vi "magnets-archive.vi"(0 "archive in":T5={"sync"={"elyse/sync/NI6071E/delay"=1.5500000000000005, "elyse/sync/NI6071E/width"=1.0, "elyse/sync/frequency/delay"=10.0, "elyse/sync/frequency/width"=181000.0, "elyse/sync/WCM/delay"=2177.9, "elyse/sync/WCM/width"=10.0, "elyse/sync/modulator/delay"=2182.400000000002, "elyse/sync/modulator/width"=3.0, "elyse/sync/HF/delay"=2175.0, "elyse/sync/HF/width"=3.0, "elyse/sync/Faraday/delay"=5080.0, "elyse/sync/Faraday/width"=100.0, "elyse/sync/Oscilloscope/delay"=2175.0, "elyse/sync/Oscilloscope/width"=2.8, "elyse/sync/50Hz_20MHz/delay"=1.0, "elyse/sync/50Hz_20MHz/width"=5000.0, "elyse/sync/laser_HF/delay"=0.35, "elyse/sync/laser_HF/width"=0.35, "elyse/sync/IMAC/delay"=2176.0, "elyse/sync/IMAC/width"=100.0, "elyse/sync/laser/delay"=2008.3, "elyse/sync/laser/width"=10.0, "elyse/sync/oscilloscope1/delay"=2175.0, "elyse/sync/oscilloscope1/width"=10.0, "elyse/sync/oscilloscope2/delay"=2175.0, "elyse/sync/oscilloscope2/width"=100.0, "elyse/sync/detection1/delay"=500.0, "elyse/sync/detection1/width"=500.0, "elyse/sync/detection1/delay"=0.3, "elyse/sync/detection2/width"=10.0, "elyse/sync/machine/delay"=2175.0, "elyse/sync/machine/width"=100.0, "elyse/sync/n_selection"=4.0}, "HT"={"elyse/HT/voltage/set_value"=6.5, "elyse/HT/voltage/value"=1.5625e-08, "elyse/HT/current/value"=0.0, "elyse/preamplifier/set_value"=1.5625e-08, "elyse/preamplifier/value"=0.0}, "HF"={"elyse/HF/attenuator/value"=-0.01903046052094623, "elyse/HF/dephaser/value"=-18.585806237727724, "elyse/HF/dephaser/value_manuel"=-78.82860725035081, "elyse/HF/canon/value"=0.0, "elyse/HF/section/value"=-18.585806237727724}, "vacuum"={"elyse/vacuum/preparation_chamber/state"=TRUE, "elyse/vacuum/preparation_chamber/measurement"=0.0, "elyse/vacuum/HF/state"=TRUE, "elyse/vacuum/HF/measurement"=0.0, "elyse/vacuum/canon/state"=TRUE, "elyse/vacuum/canon/measurement"=0.0, "elyse/vacuum/section/state"=TRUE, "elyse/vacuum/section/measurement"=0.0, "elyse/vacuum/dipole1/state"=TRUE, "elyse/vacuum/dipole1/measurement"=0.0, "elyse/vacuum/screen1/state"=TRUE, "elyse/vacuum/screen1/measurement"=0.0, "elyse/vacuum/mirror/state"=TRUE, "elyse/vacuum/mirror/measurement"=0.0, "elyse/vacuum/tpg300_section/state"=TRUE, "elyse/vacuum/tpg300_section/measurement"=0.0, "elyse/vacuum/valves/cathode/state"=FALSE, "elyse/vacuum/valves/injection/state"=FALSE}, "modulator"={"elyse/modulator/focale1/current/value"=0.0, "elyse/modulator/focale2/current/value"=0.0, "elyse/modulator/focale3/current/value"=0.0, "elyse/modulator/LAR/voltage/value"=0.0, "elyse/modulator/line_end/current/value"=0.0, "elyse/modulator/thyratron/currents/power/value"=0.0, "elyse/modulator/thyratron_reservoir/current/value"=0.0, "elyse/modulator/paramagnetization/current/value"=0.0, "elyse/modulator/thyratron/voltages/heating/value"=0.0, "elyse/modulator/thyratron/currents/heating/value"=0.0, "elyse/modulator/klystron/currents/power/value"=0.0, "elyse/modulator/klystron/voltages/power/value"=0.0, "elyse/modulator/klystron/currents/heating/value"=0.0, "elyse/modulator/klystron/voltages/heating/value"=0.0}, "cooling"={"elyse/cooling/section/temperature/set_value"=28.0, "elyse/cooling/section/temperature/measurement"=27.96142578125, "elyse/cooling/canon/temperature/set_value"=20.2, "elyse/cooling/canon/temperature/measurement"=26.69921875}, "magnets"={"elyse/magnets/focale/set_value"=0.0, "elyse/magnets/focale/value"=0.0, "elyse/magnets/phase_HF_laser/set_value"=0.0, "elyse/magnets/phase_HF_laser/value"=0.0, "elyse/magnets/dipole1/set_value"=0.0, "elyse/magnets/dipole1/value"=0.0, "elyse/magnets/dipole2/set_value"=0.0, "elyse/magnets/dipole2/value"=0.0, "elyse/magnets/Cor_H1/set_value"=0.0, "elyse/magnets/Cor_H1/value"=0.0, "elyse/magnets/Cor_V1/set_value"=0.0, "elyse/magnets/Cor_V1/value"=0.0, "elyse/magnets/Cor_H2/set_value"=0.0, "elyse/magnets/Cor_H2/value"=0.0, "elyse/magnets/Cor_V2/set_value"=0.0, "elyse/magnets/Cor_V2/value"=0.0, "elyse/magnets/Cor_H3/set_value"=0.0, "elyse/magnets/Cor_H3/value"=0.0, "elyse/magnets/Cor_V3/set_value"=-5.0, "elyse/magnets/Cor_V3/value"=0.0, "elyse/magnets/Cor_H4/set_value"=0.0, "elyse/magnets/Cor_H4/value"=0.0, "elyse/magnets/Cor_V4/set_value"=0.0, "elyse/magnets/Cor_V4/value"=0.0, "elyse/magnets/Cor_H5/set_value"=0.0, "elyse/magnets/Cor_H5/value"=0.0, "elyse/magnets/Cor_V5/set_value"=0.0, "elyse/magnets/Cor_V5/value"=0.0, "elyse/magnets/triplet1-1/set_value"=0.0, "elyse/magnets/triplet1-1/value"=0.0, "elyse/magnets/triplet1-2/set_value"=0.0, "elyse/magnets/triplet1-2/value"=0.0, "elyse/magnets/triplet2-1/set_value"=0.0, "elyse/magnets/triplet2-1/value"=0.0, "elyse/magnets/triplet2-2/set_value"=0.0, "elyse/magnets/triplet2-2/value"=0.0, "elyse/magnets/qudrupole1/set_value"=0.0, "elyse/magnets/qudrupole1/value"=0.0, "elyse/magnets/qudrupole2/set_value"=0.0, "elyse/magnets/qudrupole2/value"=0.0}, "time"={"elyse/timestamp"=0.0}}, 1 "C6NI6703":T3 {"09 OUT09 b37 Cmd Guidage V5" format="%.3f"; "08 OUT08 b33 Réserve" format="%.3f"; "07 OUT07 b29 Cmd Guidage V4" format="%.3f"; "06 OUT06 b25 Cmd Guidage H4" format="%.3f"; "05 OUT05 b21 Cmd Guidage V3" format="%.3f"; "04 OUT04 b17 Cmd Guidage H3" format="%.3f"; "03 OUT03 b13 Cmd Guidage V2" format="%.3f"; "02 OUT02 b09 Cmd Guidage H2" format="%.3f"; "01 OUT01 b05 Cmd Guidage V1" format="%.3f"; "00 OUT00 b01 Cmd Guidage H1" format="%.3f"}, 2 "C7NI6703":T2 {"09 OUT09 b37 Cmd I Dipôle 2" format="%.3f"; "08 OUT08 b33 Cmd I Dipôle 1" format="%.3f"; "07 OUT07 b29 Cmd I Quad 2" format="%.3f"; "06 OUT06 b25 Cmd I Quad 1" format="%.3f"; "05 OUT05 b21 Cmd I Solénoïde" format="%.3f"; "04 OUT04 b17 Cmd I Triplet 2-2" format="%.3f"; "03 OUT03 b13 Cmd I Triplet 2-1" format="%.3f"; "02 OUT02 b09 Réserve" format="%.3f"; "01 OUT01 b05 Cmd I Triplet 1-2" format="%.3f"; "00 OUT00 b01 Cmd I Triplet 1-1" format="%.3f"}, 3 "C8NI6703":T4 {"09 OUT09 b37 Cmd position Miroir Y" format="%.3f"; "08 OUT08 b33 Cmd position Miroir X" format="%.3f"; "07 OUT07 b29 Réserve" format="%.3f"; "06 OUT06 b25 Cmd amplitude HF préampli" format="%.3f"; "05 OUT05 b21 Cmd déphasage HF/LASER" format="%.3f"; "04 OUT04 b17 Cmd Pos. Atténuateur" format="%.3f"; "03 OUT03 b13 Cmd Pos. Déphaseur" format="%.3f"; "02 OUT02 b09 Cmd Temp. Section" format="%.3f"; "01 OUT01 b05 Cmd Temp. Canon" format="%.3f"; "00 OUT00 b01 Réserve" format="%.3f"}, 4 "C1NI6071E":T1 {"63 ACH63 b100 Libre ?" format="%.3f"; "62 ACH62 b98 Libre ?" format="%.3f"; "61 ACH61 b96 Libre ?" format="%.3f"; "60 ACH60 b94 Libre ?" format="%.3f"; "59 ACH59 b92 Libre ?" format="%.3f"; "58 ACH58 b90 Libre ?" format="%.3f"; "57 ACH57 b88 Libre ?" format="%.3f"; "56 ACH56 b86 Libre ?" format="%.3f"; "55 ACH55 b99 Libre ?" format="%.3f"; "54 ACH54 b97 Libre ?" format="%.3f"; "53 ACH53 b95 Libre ?" format="%.3f"; "52 ACH52 b93 Libre ?" format="%.3f"; "51 ACH51 b91 Libre ?" format="%.3f"; "50 ACH50 b89 Libre ?" format="%.3f"; "49 ACH49 b87 Libre ?" format="%.3f"; "48 ACH48 b85 Réservé" format="%.3f"; "47 ACH47 b84 Réservé" format="%.3f"; "46 ACH46 b82 Réservé" format="%.3f"; "45 ACH45 b80 Mesure phase HF1" format="%.3f"; "44 ACH44 b78 Mesure Atténuateur" format="%.3f"; "43 ACH43 b74 Réservé" format="%.3f"; "42 ACH42 b72 Mes champ Dipôle 2" format="%.3f"; "41 ACH41 b70 Mes H5" format="%.3f"; "40 ACH40 b68 Mes I correcte Dipôle 21 (H4)" format="%.3f"; "39 ACH39 b83 Réservé" format="%.3f"; "38 ACH38 b81 Mesure phase HF2" format="%.3f"; "37 ACH37 b79 Mes position Déphaseur ajust" format="%.3f"; "36 ACH36 b77 Mes position Déphaseur" format="%.3f"; "35 ACH35 b73 Mes champ Dipôle 2" format="%.3f"; "34 ACH34 b71 Mes I Guidage V5" format="%.3f"; "33 ACH33 b69 Mes I Guidage V4" format="%.3f"; "32 ACH32 b67 Mes I Guidage V3" format="%.3f"; "31 ACH31 b66 Mes I correcte Dipôle 1 (H3)" format="%.3f"; "30 ACH30 b64 Mes I Guidage H2" format="%.3f"; "29 ACH29 b62 Mes I Guidage H1" format="%.3f"; "28 ACH28 b60 Mes I Dipôle 1" format="%.3f"; "27 ACH27 b58 Mes I Quadripôle 2" format="%.3f"; "26 ACH26 b56 Réservé" format="%.3f"; "25 ACH25 b54 Mes I Triplet 2-1" format="%.3f"; "24 ACH24 b52 Mes I Triplet 1-2" format="%.3f"; "23 ACH23 b65 Mes I Guidage V2" format="%.3f"; "22 ACH22 b63 Mes I Guidage V1" format="%.3f"; "21 ACH21 b61 Mes I Dipôle 2" format="%.3f"; "20 ACH20 b59 Mes I Solénoïde" format="%.3f"; "19 ACH19 b57 Mes I Quadripôle 1" format="%.3f"; "18 ACH18 b55 Mes I Triplet 2-2" format="%.3f"; "17 ACH17 b53 Réservé" format="%.3f"; "16 ACH16 b51 Mes I Triplet 1-1" format="%.3f"; "15 ACH15 b18 Libre ?" format="%.3f"; "14 ACH14 b16 Libre ?" format="%.3f"; "13 ACH13 b14 Libre ?" format="%.3f"; "12 ACH12 b12 Mes Vide jauge canon" format="%.3f"; "11 ACH11 b10 Mes Vide DIP 1 (PIQ27 + 33)" format="%.3f"; "10 ACH10 b08 Mes Vide Section (PIQ 16)" format="%.3f"; "09 ACH09 b06 Mes Vide SAS guide HF" format="%.3f"; "08 ACH08 b04 Mes température Section" format="%.3f"; "07 ACH07 b17 Libre ?" format="%.3f"; "06 ACH06 b15 Libre ?" format="%.3f"; "05 ACH05 b13 Libre ?" format="%.3f"; "04 ACH04 b11 Mes Vide Ecran 1 (PIQ 53-63)" format="%.3f"; "03 ACH03 b09 Mes Vide Miroir (PIQ 21)" format="%.3f"; "02 ACH02 b07 Mes Vide Canon (PIQ 12)" format="%.3f"; "01 ACH01 b05 Mes Vide Chambre de préparation" format="%.3f"; "00 ACH00 b03 Mes température Canon" format="%.3f"}) -> (5 "archive out":T5={"sync"={"elyse/sync/NI6071E/delay"=1.5500000000000005, "elyse/sync/NI6071E/width"=1.0, "elyse/sync/frequency/delay"=10.0, "elyse/sync/frequency/width"=181000.0, "elyse/sync/WCM/delay"=2177.9, "elyse/sync/WCM/width"=10.0, "elyse/sync/modulator/delay"=2182.400000000002, "elyse/sync/modulator/width"=3.0, "elyse/sync/HF/delay"=2175.0, "elyse/sync/HF/width"=3.0, "elyse/sync/Faraday/delay"=5080.0, "elyse/sync/Faraday/width"=100.0, "elyse/sync/Oscilloscope/delay"=2175.0, "elyse/sync/Oscilloscope/width"=2.8, "elyse/sync/50Hz_20MHz/delay"=1.0, "elyse/sync/50Hz_20MHz/width"=5000.0, "elyse/sync/laser_HF/delay"=0.35, "elyse/sync/laser_HF/width"=0.35, "elyse/sync/IMAC/delay"=2176.0, "elyse/sync/IMAC/width"=100.0, "elyse/sync/laser/delay"=2008.3, "elyse/sync/laser/width"=10.0, "elyse/sync/oscilloscope1/delay"=2175.0, "elyse/sync/oscilloscope1/width"=10.0, "elyse/sync/oscilloscope2/delay"=2175.0, "elyse/sync/oscilloscope2/width"=100.0, "elyse/sync/detection1/delay"=500.0, "elyse/sync/detection1/width"=500.0, "elyse/sync/detection1/delay"=0.3, "elyse/sync/detection2/width"=10.0, "elyse/sync/machine/delay"=2175.0, "elyse/sync/machine/width"=100.0, "elyse/sync/n_selection"=4.0}, "HT"={"elyse/HT/voltage/set_value"=6.5, "elyse/HT/voltage/value"=1.5625e-08, "elyse/HT/current/value"=0.0, "elyse/preamplifier/set_value"=1.5625e-08, "elyse/preamplifier/value"=0.0}, "HF"={"elyse/HF/attenuator/value"=-0.01903046052094623, "elyse/HF/dephaser/value"=-18.585806237727724, "elyse/HF/dephaser/value_manuel"=-78.82860725035081, "elyse/HF/canon/value"=0.0, "elyse/HF/section/value"=-18.585806237727724}, "vacuum"={"elyse/vacuum/preparation_chamber/state"=TRUE, "elyse/vacuum/preparation_chamber/measurement"=0.0, "elyse/vacuum/HF/state"=TRUE, "elyse/vacuum/HF/measurement"=0.0, "elyse/vacuum/canon/state"=TRUE, "elyse/vacuum/canon/measurement"=0.0, "elyse/vacuum/section/state"=TRUE, "elyse/vacuum/section/measurement"=0.0, "elyse/vacuum/dipole1/state"=TRUE, "elyse/vacuum/dipole1/measurement"=0.0, "elyse/vacuum/screen1/state"=TRUE, "elyse/vacuum/screen1/measurement"=0.0, "elyse/vacuum/mirror/state"=TRUE, "elyse/vacuum/mirror/measurement"=0.0, "elyse/vacuum/tpg300_section/state"=TRUE, "elyse/vacuum/tpg300_section/measurement"=0.0, "elyse/vacuum/valves/cathode/state"=FALSE, "elyse/vacuum/valves/injection/state"=FALSE}, "modulator"={"elyse/modulator/focale1/current/value"=0.0, "elyse/modulator/focale2/current/value"=0.0, "elyse/modulator/focale3/current/value"=0.0, "elyse/modulator/LAR/voltage/value"=0.0, "elyse/modulator/line_end/current/value"=0.0, "elyse/modulator/thyratron/currents/power/value"=0.0, "elyse/modulator/thyratron_reservoir/current/value"=0.0, "elyse/modulator/paramagnetization/current/value"=0.0, "elyse/modulator/thyratron/voltages/heating/value"=0.0, "elyse/modulator/thyratron/currents/heating/value"=0.0, "elyse/modulator/klystron/currents/power/value"=0.0, "elyse/modulator/klystron/voltages/power/value"=0.0, "elyse/modulator/klystron/currents/heating/value"=0.0, "elyse/modulator/klystron/voltages/heating/value"=0.0}, "cooling"={"elyse/cooling/section/temperature/set_value"=28.0, "elyse/cooling/section/temperature/measurement"=27.96142578125, "elyse/cooling/canon/temperature/set_value"=20.2, "elyse/cooling/canon/temperature/measurement"=26.69921875}, "magnets"={"elyse/magnets/focale/set_value"=0.0, "elyse/magnets/focale/value"=0.0, "elyse/magnets/phase_HF_laser/set_value"=0.0, "elyse/magnets/phase_HF_laser/value"=0.0, "elyse/magnets/dipole1/set_value"=0.0, "elyse/magnets/dipole1/value"=0.0, "elyse/magnets/dipole2/set_value"=0.0, "elyse/magnets/dipole2/value"=0.0, "elyse/magnets/Cor_H1/set_value"=0.0, "elyse/magnets/Cor_H1/value"=0.0, "elyse/magnets/Cor_V1/set_value"=0.0, "elyse/magnets/Cor_V1/value"=0.0, "elyse/magnets/Cor_H2/set_value"=0.0, "elyse/magnets/Cor_H2/value"=0.0, "elyse/magnets/Cor_V2/set_value"=0.0, "elyse/magnets/Cor_V2/value"=0.0, "elyse/magnets/Cor_H3/set_value"=0.0, "elyse/magnets/Cor_H3/value"=0.0, "elyse/magnets/Cor_V3/set_value"=-5.0, "elyse/magnets/Cor_V3/value"=0.0, "elyse/magnets/Cor_H4/set_value"=0.0, "elyse/magnets/Cor_H4/value"=0.0, "elyse/magnets/Cor_V4/set_value"=0.0, "elyse/magnets/Cor_V4/value"=0.0, "elyse/magnets/Cor_H5/set_value"=0.0, "elyse/magnets/Cor_H5/value"=0.0, "elyse/magnets/Cor_V5/set_value"=0.0, "elyse/magnets/Cor_V5/value"=0.0, "elyse/magnets/triplet1-1/set_value"=0.0, "elyse/magnets/triplet1-1/value"=0.0, "elyse/magnets/triplet1-2/set_value"=0.0, "elyse/magnets/triplet1-2/value"=0.0, "elyse/magnets/triplet2-1/set_value"=0.0, "elyse/magnets/triplet2-1/value"=0.0, "elyse/magnets/triplet2-2/set_value"=0.0, "elyse/magnets/triplet2-2/value"=0.0, "elyse/magnets/qudrupole1/set_value"=0.0, "elyse/magnets/qudrupole1/value"=0.0, "elyse/magnets/qudrupole2/set_value"=0.0, "elyse/magnets/qudrupole2/value"=0.0}, "time"={"elyse/timestamp"=0.0}})   [LabVIEW 2020]
uses:
  archive.ctl
  sync_type_def.ctl
  HT_type-def.ctl
  HF_type_def.ctl
  vacuum_type_def.ctl
  modulator_type_def.ctl
  water_cooling_type_def.ctl
  all_magnets_type_def.ctl
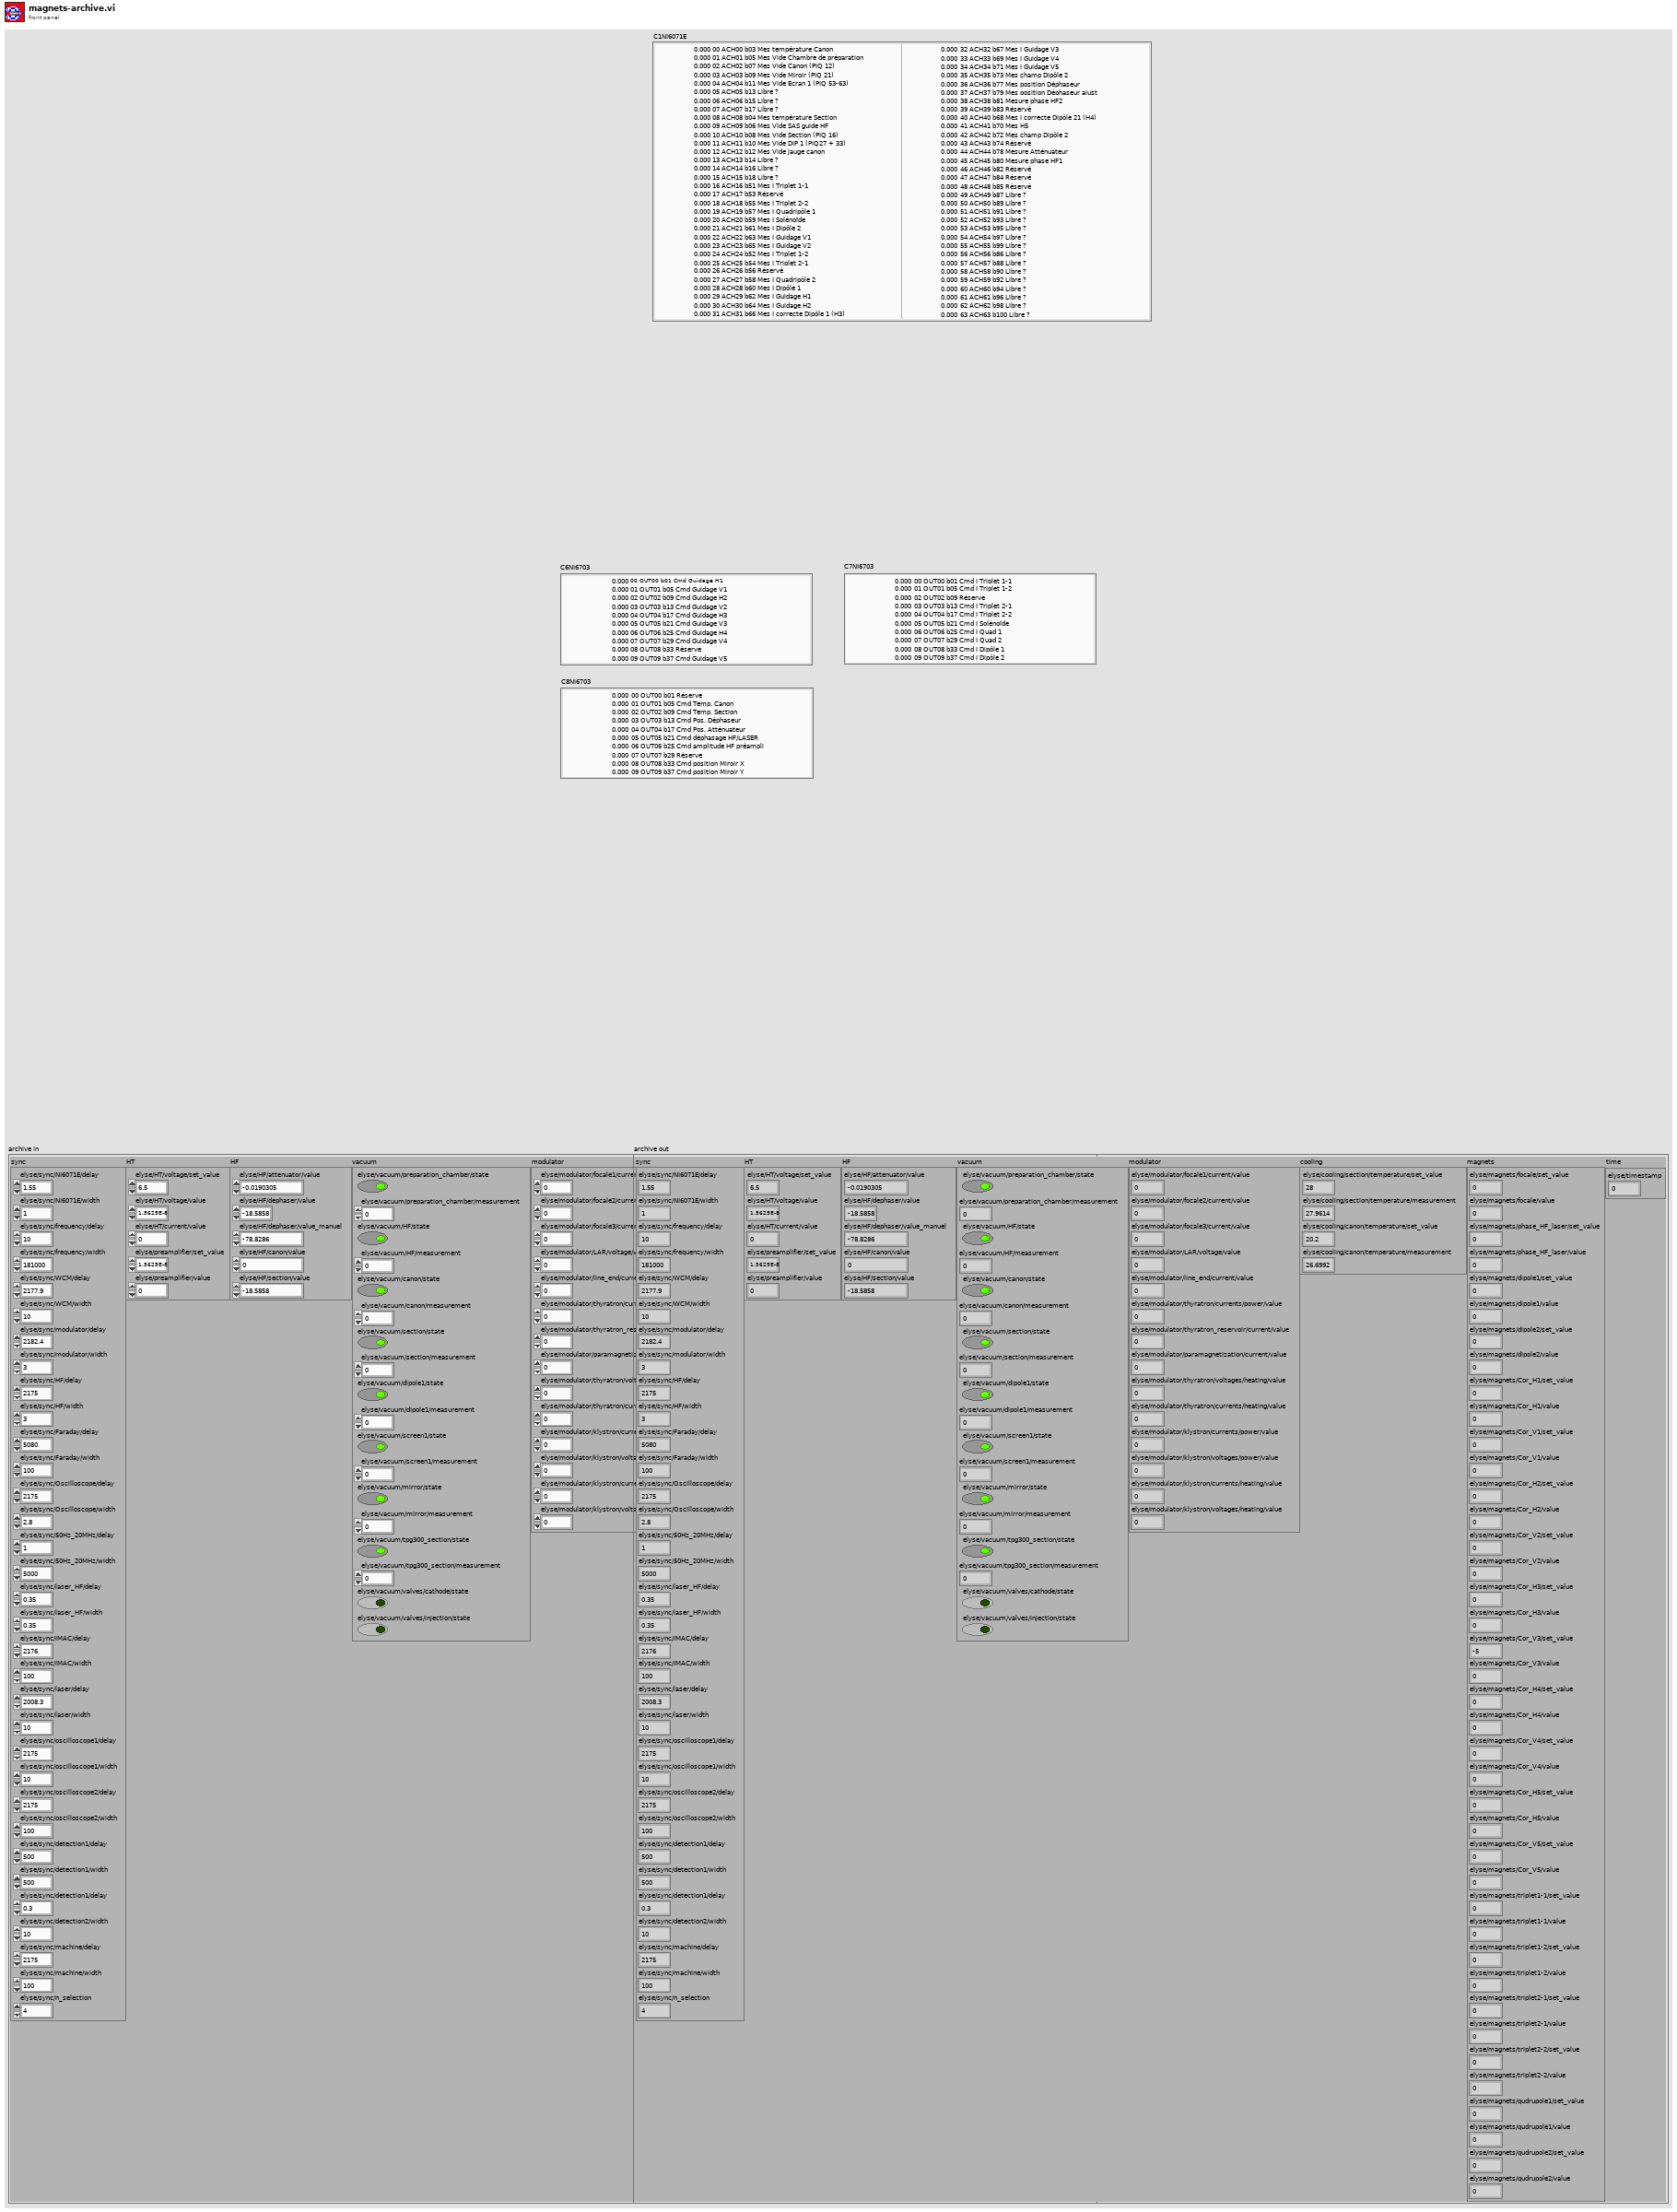
[diagram p1: front panel]
types:
  T1 = cluster{"00 ACH00 b03 Mes température Canon":dbl, "01 ACH01 b05 Mes Vide Chambre de préparation":dbl, "02 ACH02 b07 Mes Vide Canon (PIQ 12)":dbl, "03 ACH03 b09 Mes Vide Miroir (PIQ 21)":dbl, "04 ACH04 b11 Mes Vide Ecran 1 (PIQ 53-63)":dbl, "05 ACH05 b13 Libre ?":dbl, "06 ACH06 b15 Libre ?":dbl, "07 ACH07 b17 Libre ?":dbl, "08 ACH08 b04 Mes température Section":dbl, "09 ACH09 b06 Mes Vide SAS guide HF":dbl, "10 ACH10 b08 Mes Vide Section (PIQ 16)":dbl, "11 ACH11 b10 Mes Vide DIP 1 (PIQ27 + 33)":dbl, "12 ACH12 b12 Mes Vide jauge canon":dbl, "13 ACH13 b14 Libre ?":dbl, "14 ACH14 b16 Libre ?":dbl, "15 ACH15 b18 Libre ?":dbl, "16 ACH16 b51 Mes I Triplet 1-1":dbl, "17 ACH17 b53 Réservé":dbl, "18 ACH18 b55 Mes I Triplet 2-2":dbl, "19 ACH19 b57 Mes I Quadripôle 1":dbl, "20 ACH20 b59 Mes I Solénoïde":dbl, "21 ACH21 b61 Mes I Dipôle 2":dbl, "22 ACH22 b63 Mes I Guidage V1":dbl, "23 ACH23 b65 Mes I Guidage V2":dbl, "24 ACH24 b52 Mes I Triplet 1-2":dbl, "25 ACH25 b54 Mes I Triplet 2-1":dbl, "26 ACH26 b56 Réservé":dbl, "27 ACH27 b58 Mes I Quadripôle 2":dbl, "28 ACH28 b60 Mes I Dipôle 1":dbl, "29 ACH29 b62 Mes I Guidage H1":dbl, "30 ACH30 b64 Mes I Guidage H2":dbl, "31 ACH31 b66 Mes I correcte Dipôle 1 (H3)":dbl, "32 ACH32 b67 Mes I Guidage V3":dbl, "33 ACH33 b69 Mes I Guidage V4":dbl, "34 ACH34 b71 Mes I Guidage V5":dbl, "35 ACH35 b73 Mes champ Dipôle 2":dbl, "36 ACH36 b77 Mes position Déphaseur":dbl, "37 ACH37 b79 Mes position Déphaseur ajust":dbl, "38 ACH38 b81 Mesure phase HF2":dbl, "39 ACH39 b83 Réservé":dbl, "40 ACH40 b68 Mes I correcte Dipôle 21 (H4)":dbl, "41 ACH41 b70 Mes H5":dbl, "42 ACH42 b72 Mes champ Dipôle 2":dbl, "43 ACH43 b74 Réservé":dbl, "44 ACH44 b78 Mesure Atténuateur":dbl, "45 ACH45 b80 Mesure phase HF1":dbl, "46 ACH46 b82 Réservé":dbl, "47 ACH47 b84 Réservé":dbl, "48 ACH48 b85 Réservé":dbl, "49 ACH49 b87 Libre ?":dbl, "50 ACH50 b89 Libre ?":dbl, "51 ACH51 b91 Libre ?":dbl, "52 ACH52 b93 Libre ?":dbl, "53 ACH53 b95 Libre ?":dbl, "54 ACH54 b97 Libre ?":dbl, "55 ACH55 b99 Libre ?":dbl, "56 ACH56 b86 Libre ?":dbl, "57 ACH57 b88 Libre ?":dbl, "58 ACH58 b90 Libre ?":dbl, "59 ACH59 b92 Libre ?":dbl, "60 ACH60 b94 Libre ?":dbl, "61 ACH61 b96 Libre ?":dbl, "62 ACH62 b98 Libre ?":dbl, "63 ACH63 b100 Libre ?":dbl}
  T2 = cluster{"00 OUT00 b01 Cmd I Triplet 1-1":dbl, "01 OUT01 b05 Cmd I Triplet 1-2":dbl, "02 OUT02 b09 Réserve":dbl, "03 OUT03 b13 Cmd I Triplet 2-1":dbl, "04 OUT04 b17 Cmd I Triplet 2-2":dbl, "05 OUT05 b21 Cmd I Solénoïde":dbl, "06 OUT06 b25 Cmd I Quad 1":dbl, "07 OUT07 b29 Cmd I Quad 2":dbl, "08 OUT08 b33 Cmd I Dipôle 1":dbl, "09 OUT09 b37 Cmd I Dipôle 2":dbl}
  T3 = cluster{"00 OUT00 b01 Cmd Guidage H1":dbl, "01 OUT01 b05 Cmd Guidage V1":dbl, "02 OUT02 b09 Cmd Guidage H2":dbl, "03 OUT03 b13 Cmd Guidage V2":dbl, "04 OUT04 b17 Cmd Guidage H3":dbl, "05 OUT05 b21 Cmd Guidage V3":dbl, "06 OUT06 b25 Cmd Guidage H4":dbl, "07 OUT07 b29 Cmd Guidage V4":dbl, "08 OUT08 b33 Réserve":dbl, "09 OUT09 b37 Cmd Guidage V5":dbl}
  T4 = cluster{"00 OUT00 b01 Réserve":dbl, "01 OUT01 b05 Cmd Temp. Canon":dbl, "02 OUT02 b09 Cmd Temp. Section":dbl, "03 OUT03 b13 Cmd Pos. Déphaseur":dbl, "04 OUT04 b17 Cmd Pos. Atténuateur":dbl, "05 OUT05 b21 Cmd déphasage HF/LASER":dbl, "06 OUT06 b25 Cmd amplitude HF préampli":dbl, "07 OUT07 b29 Réserve":dbl, "08 OUT08 b33 Cmd position Miroir X":dbl, "09 OUT09 b37 Cmd position Miroir Y":dbl}
  T5 = typedef "archive.ctl" = cluster{"sync":T6, "HT":T7, "HF":T8, "vacuum":T9, "modulator":T10, "cooling":T11, "magnets":T12, "time":cluster{"elyse/timestamp":dbl}}
  T6 = typedef "sync_type_def.ctl" = cluster{"elyse/sync/NI6071E/delay":dbl, "elyse/sync/NI6071E/width":dbl, "elyse/sync/frequency/delay":dbl, "elyse/sync/frequency/width":dbl, "elyse/sync/WCM/delay":dbl, "elyse/sync/WCM/width":dbl, "elyse/sync/modulator/delay":dbl, "elyse/sync/modulator/width":dbl, "elyse/sync/HF/delay":dbl, "elyse/sync/HF/width":dbl, "elyse/sync/Faraday/delay":dbl, "elyse/sync/Faraday/width":dbl, "elyse/sync/Oscilloscope/delay":dbl, "elyse/sync/Oscilloscope/width":dbl, "elyse/sync/50Hz_20MHz/delay":dbl, "elyse/sync/50Hz_20MHz/width":dbl, "elyse/sync/laser_HF/delay":dbl, "elyse/sync/laser_HF/width":dbl, "elyse/sync/IMAC/delay":dbl, "elyse/sync/IMAC/width":dbl, "elyse/sync/laser/delay":dbl, "elyse/sync/laser/width":dbl, "elyse/sync/oscilloscope1/delay":dbl, "elyse/sync/oscilloscope1/width":dbl, "elyse/sync/oscilloscope2/delay":dbl, "elyse/sync/oscilloscope2/width":dbl, "elyse/sync/detection1/delay":dbl, "elyse/sync/detection1/width":dbl, "elyse/sync/detection1/delay":dbl, "elyse/sync/detection2/width":dbl, "elyse/sync/machine/delay":dbl, "elyse/sync/machine/width":dbl, "elyse/sync/n_selection":dbl}
  T7 = typedef "HT_type-def.ctl" = cluster{"elyse/HT/voltage/set_value":dbl, "elyse/HT/voltage/value":dbl, "elyse/HT/current/value":dbl, "elyse/preamplifier/set_value":dbl, "elyse/preamplifier/value":dbl}
  T8 = typedef "HF_type_def.ctl" = cluster{"elyse/HF/attenuator/value":dbl, "elyse/HF/dephaser/value":dbl, "elyse/HF/dephaser/value_manuel":dbl, "elyse/HF/canon/value":dbl, "elyse/HF/section/value":dbl}
  T9 = typedef "vacuum_type_def.ctl" = cluster{"elyse/vacuum/preparation_chamber/state":bool, "elyse/vacuum/preparation_chamber/measurement":dbl, "elyse/vacuum/HF/state":bool, "elyse/vacuum/HF/measurement":dbl, "elyse/vacuum/canon/state":bool, "elyse/vacuum/canon/measurement":dbl, "elyse/vacuum/section/state":bool, "elyse/vacuum/section/measurement":dbl, "elyse/vacuum/dipole1/state":bool, "elyse/vacuum/dipole1/measurement":dbl, "elyse/vacuum/screen1/state":bool, "elyse/vacuum/screen1/measurement":dbl, "elyse/vacuum/mirror/state":bool, "elyse/vacuum/mirror/measurement":dbl, "elyse/vacuum/tpg300_section/state":bool, "elyse/vacuum/tpg300_section/measurement":dbl, "elyse/vacuum/valves/cathode/state":bool, "elyse/vacuum/valves/injection/state":bool}
  T10 = typedef "modulator_type_def.ctl" = cluster{"elyse/modulator/focale1/current/value":dbl, "elyse/modulator/focale2/current/value":dbl, "elyse/modulator/focale3/current/value":dbl, "elyse/modulator/LAR/voltage/value":dbl, "elyse/modulator/line_end/current/value":dbl, "elyse/modulator/thyratron/currents/power/value":dbl, "elyse/modulator/thyratron_reservoir/current/value":dbl, "elyse/modulator/paramagnetization/current/value":dbl, "elyse/modulator/thyratron/voltages/heating/value":dbl, "elyse/modulator/thyratron/currents/heating/value":dbl, "elyse/modulator/klystron/currents/power/value":dbl, "elyse/modulator/klystron/voltages/power/value":dbl, "elyse/modulator/klystron/currents/heating/value":dbl, "elyse/modulator/klystron/voltages/heating/value":dbl}
  T11 = typedef "water_cooling_type_def.ctl" = cluster{"elyse/cooling/section/temperature/set_value":dbl, "elyse/cooling/section/temperature/measurement":dbl, "elyse/cooling/canon/temperature/set_value":dbl, "elyse/cooling/canon/temperature/measurement":dbl}
  T12 = typedef "all_magnets_type_def.ctl" = cluster{"elyse/magnets/focale/set_value":dbl, "elyse/magnets/focale/value":dbl, "elyse/magnets/phase_HF_laser/set_value":dbl, "elyse/magnets/phase_HF_laser/value":dbl, "elyse/magnets/dipole1/set_value":dbl, "elyse/magnets/dipole1/value":dbl, "elyse/magnets/dipole2/set_value":dbl, "elyse/magnets/dipole2/value":dbl, "elyse/magnets/Cor_H1/set_value":dbl, "elyse/magnets/Cor_H1/value":dbl, "elyse/magnets/Cor_V1/set_value":dbl, "elyse/magnets/Cor_V1/value":dbl, "elyse/magnets/Cor_H2/set_value":dbl, "elyse/magnets/Cor_H2/value":dbl, "elyse/magnets/Cor_V2/set_value":dbl, "elyse/magnets/Cor_V2/value":dbl, "elyse/magnets/Cor_H3/set_value":dbl, "elyse/magnets/Cor_H3/value":dbl, "elyse/magnets/Cor_V3/set_value":dbl, "elyse/magnets/Cor_V3/value":dbl, "elyse/magnets/Cor_H4/set_value":dbl, "elyse/magnets/Cor_H4/value":dbl, "elyse/magnets/Cor_V4/set_value":dbl, "elyse/magnets/Cor_V4/value":dbl, "elyse/magnets/Cor_H5/set_value":dbl, "elyse/magnets/Cor_H5/value":dbl, "elyse/magnets/Cor_V5/set_value":dbl, "elyse/magnets/Cor_V5/value":dbl, "elyse/magnets/triplet1-1/set_value":dbl, "elyse/magnets/triplet1-1/value":dbl, "elyse/magnets/triplet1-2/set_value":dbl, "elyse/magnets/triplet1-2/value":dbl, "elyse/magnets/triplet2-1/set_value":dbl, "elyse/magnets/triplet2-1/value":dbl, "elyse/magnets/triplet2-2/set_value":dbl, "elyse/magnets/triplet2-2/value":dbl, "elyse/magnets/qudrupole1/set_value":dbl, "elyse/magnets/qudrupole1/value":dbl, "elyse/magnets/qudrupole2/set_value":dbl, "elyse/magnets/qudrupole2/value":dbl}
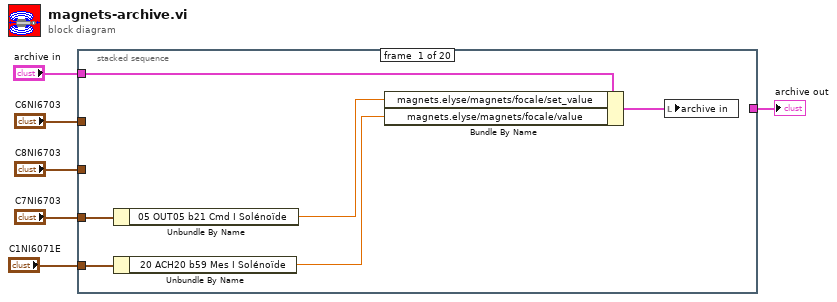
[diagram p0: block diagram]
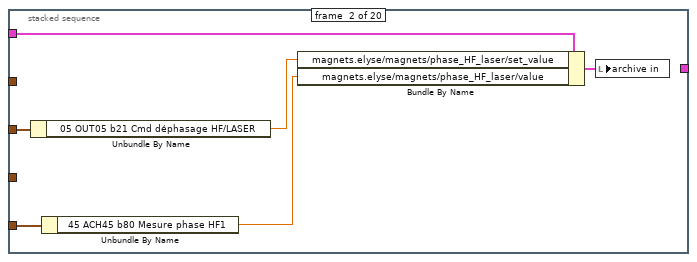
[diagram p2: hidden frame]
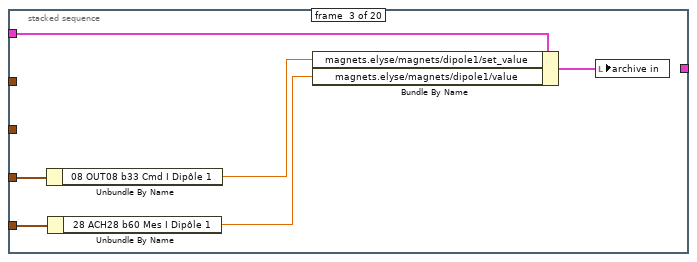
[diagram p3: hidden frame]
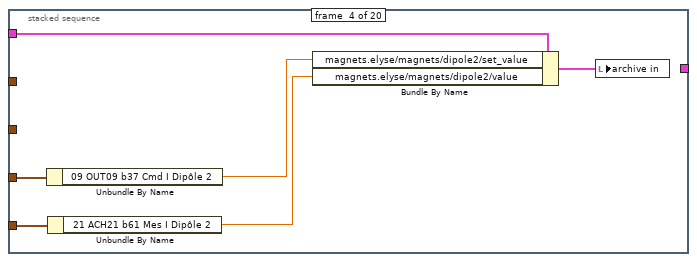
[diagram p4: hidden frame]
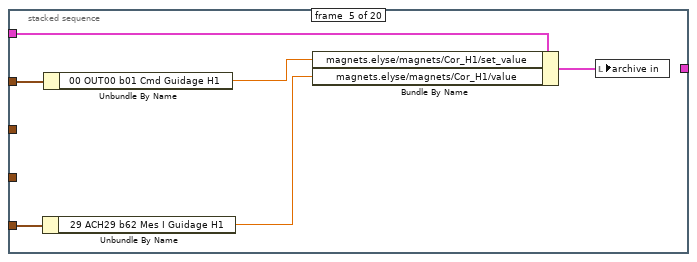
[diagram p5: hidden frame]
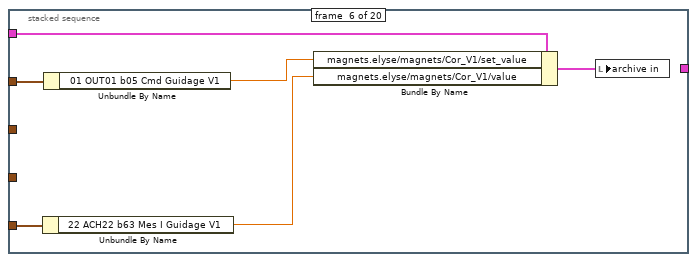
[diagram p6: hidden frame]
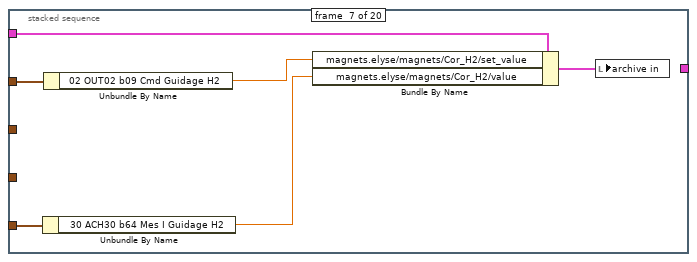
[diagram p7: hidden frame]
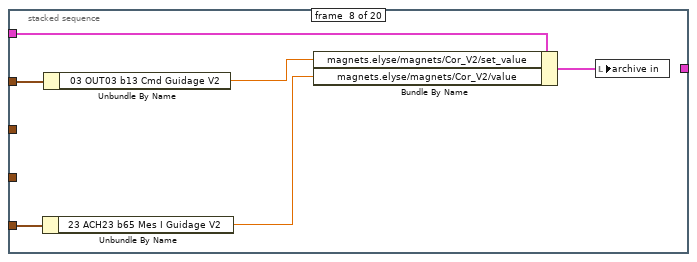
[diagram p8: hidden frame]
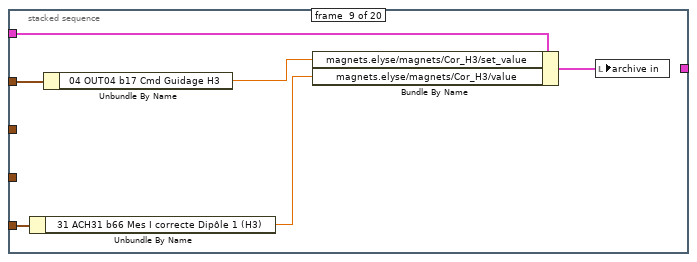
[diagram p9: hidden frame]
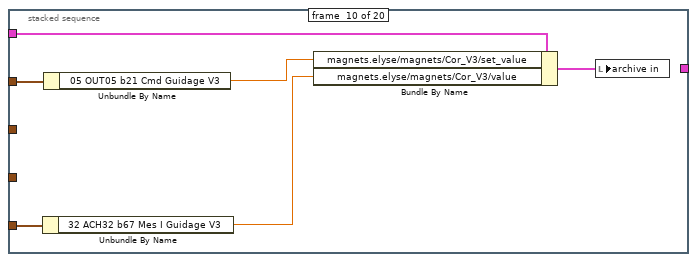
[diagram p10: hidden frame]
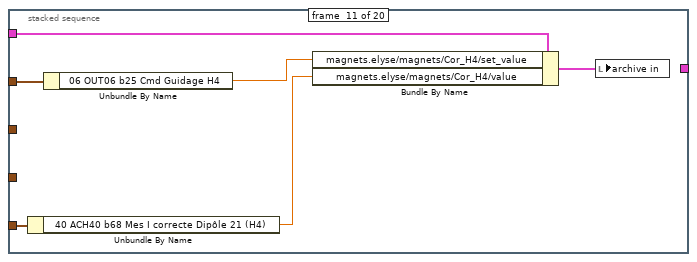
[diagram p11: hidden frame]
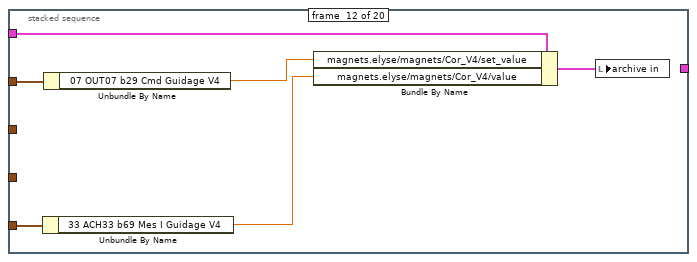
[diagram p12: hidden frame]
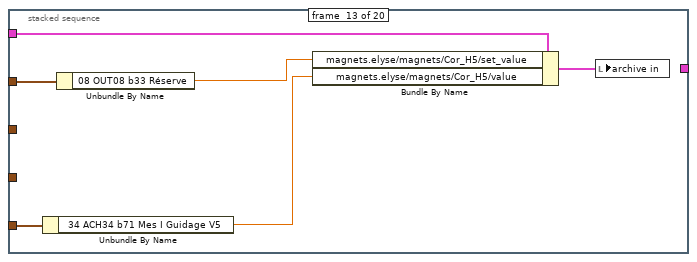
[diagram p13: hidden frame]
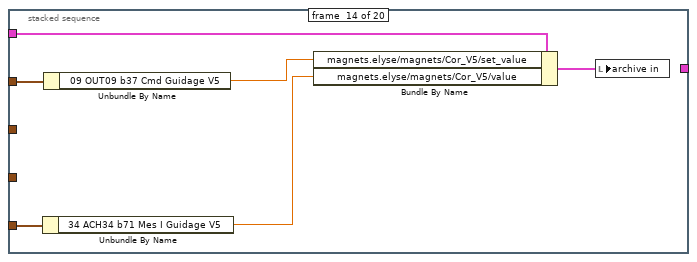
[diagram p14: hidden frame]
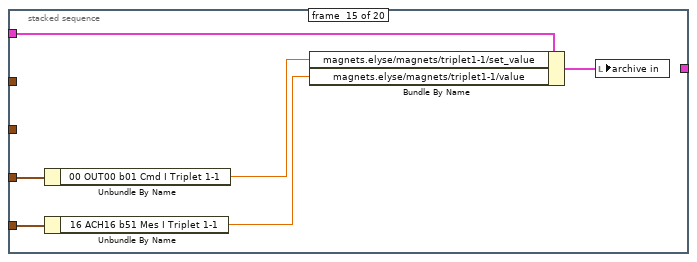
[diagram p15: hidden frame]
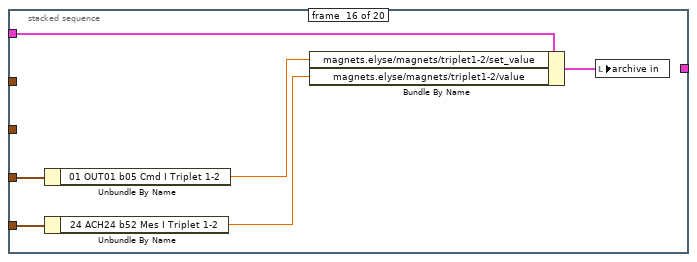
[diagram p16: hidden frame]
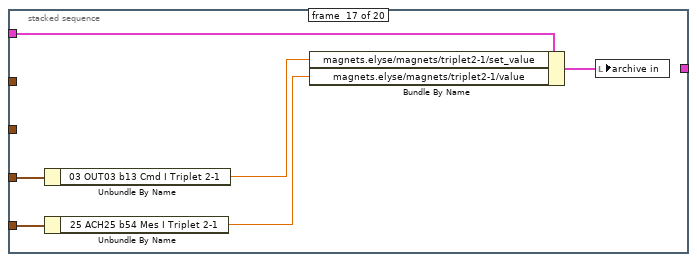
[diagram p17: hidden frame]
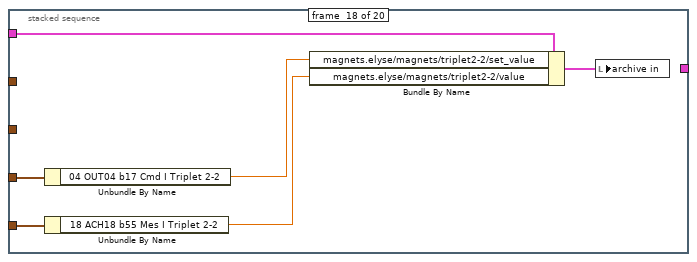
[diagram p18: hidden frame]
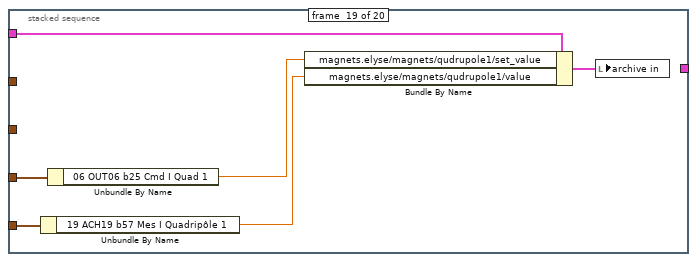
[diagram p19: hidden frame]
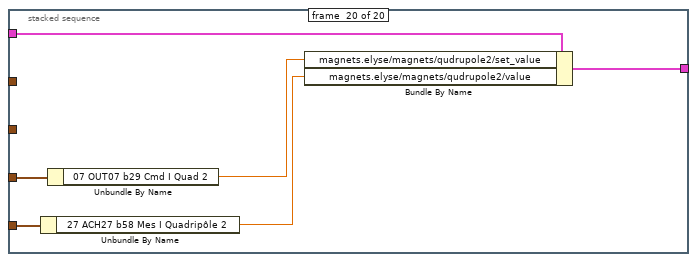
[diagram p20: hidden frame]
diagram:
  n1 = stacked-sequence {
    tunnel: "archive in" -> [w8 w14 w20 w26 w32 w38 w44 w50 w56 w62 w68 w74 w80 w86 w92 w98 w104 w110 w116 w122]
    tunnel: "C1NI6071E" -> [w11 w17 w23 w29 w35 w41 w47 w54 w60 w66 w72 w78 w84 w87 w96 w101 w108 w112 w120 w126]
    tunnel: "C6NI6703" -> [_ _ _ _ w34 w40 w46 w52 w58 w64 w70 w76 w82 w89 _ _ _ _ _ _]
    tunnel: "C7NI6703" -> [w10 _ w22 w28 _ _ _ _ _ _ _ _ _ _ w93 w99 w107 w114 w118 w124]
    tunnel: "C8NI6703" -> [_ w16 _ _ _ _ _ _ _ _ _ _ _ _ _ _ _ _ _ _]
    tunnel: [_ _ _ _ _ _ _ _ _ _ _ _ _ _ _ _ _ _ _ w121] -> w1
    frame #0 {
      n2 = Unbundle By Name(w10) -> ("05 OUT05 b21 Cmd I Solénoïde"=w9:dbl)
      n3 = Unbundle By Name(w11) -> ("20 ACH20 b59 Mes I Solénoïde"=w12:dbl)
      n4 = Bundle By Name(cluster=w8, "magnets.elyse/magnets/focale/set_value"=w9, "magnets.elyse/magnets/focale/value"=w12) -> (w7:T5)
      n5 = local write "archive in"(w7) -> ()
    }
    frame #1 {
      n6 = Unbundle By Name(w16) -> ("05 OUT05 b21 Cmd déphasage HF/LASER"=w15:dbl)
      n7 = Unbundle By Name(w17) -> ("45 ACH45 b80 Mesure phase HF1"=w18:dbl)
      n8 = Bundle By Name(cluster=w14, "magnets.elyse/magnets/phase_HF_laser/set_value"=w15, "magnets.elyse/magnets/phase_HF_laser/value"=w18) -> (w13:T5)
      n9 = local write "archive in"(w13) -> ()
    }
    frame #2 {
      n10 = Unbundle By Name(w22) -> ("08 OUT08 b33 Cmd I Dipôle 1"=w21:dbl)
      n11 = Unbundle By Name(w23) -> ("28 ACH28 b60 Mes I Dipôle 1"=w24:dbl)
      n12 = Bundle By Name(cluster=w20, "magnets.elyse/magnets/dipole1/set_value"=w21, "magnets.elyse/magnets/dipole1/value"=w24) -> (w19:T5)
      n13 = local write "archive in"(w19) -> ()
    }
    frame #3 {
      n14 = Unbundle By Name(w28) -> ("09 OUT09 b37 Cmd I Dipôle 2"=w27:dbl)
      n15 = Unbundle By Name(w29) -> ("21 ACH21 b61 Mes I Dipôle 2"=w30:dbl)
      n16 = Bundle By Name(cluster=w26, "magnets.elyse/magnets/dipole2/set_value"=w27, "magnets.elyse/magnets/dipole2/value"=w30) -> (w25:T5)
      n17 = local write "archive in"(w25) -> ()
    }
    frame #4 {
      n18 = Unbundle By Name(w35) -> ("29 ACH29 b62 Mes I Guidage H1"=w36:dbl)
      n19 = Unbundle By Name(w34) -> ("00 OUT00 b01 Cmd Guidage H1"=w33:dbl)
      n20 = Bundle By Name(cluster=w32, "magnets.elyse/magnets/Cor_H1/set_value"=w33, "magnets.elyse/magnets/Cor_H1/value"=w36) -> (w31:T5)
      n21 = local write "archive in"(w31) -> ()
    }
    frame #5 {
      n22 = Unbundle By Name(w41) -> ("22 ACH22 b63 Mes I Guidage V1"=w42:dbl)
      n23 = Unbundle By Name(w40) -> ("01 OUT01 b05 Cmd Guidage V1"=w39:dbl)
      n24 = Bundle By Name(cluster=w38, "magnets.elyse/magnets/Cor_V1/set_value"=w39, "magnets.elyse/magnets/Cor_V1/value"=w42) -> (w37:T5)
      n25 = local write "archive in"(w37) -> ()
    }
    frame #6 {
      n26 = Unbundle By Name(w47) -> ("30 ACH30 b64 Mes I Guidage H2"=w48:dbl)
      n27 = Unbundle By Name(w46) -> ("02 OUT02 b09 Cmd Guidage H2"=w45:dbl)
      n28 = Bundle By Name(cluster=w44, "magnets.elyse/magnets/Cor_H2/set_value"=w45, "magnets.elyse/magnets/Cor_H2/value"=w48) -> (w43:T5)
      n29 = local write "archive in"(w43) -> ()
    }
    frame #7 {
      n30 = Unbundle By Name(w54) -> ("23 ACH23 b65 Mes I Guidage V2"=w53:dbl)
      n31 = Unbundle By Name(w52) -> ("03 OUT03 b13 Cmd Guidage V2"=w51:dbl)
      n32 = Bundle By Name(cluster=w50, "magnets.elyse/magnets/Cor_V2/set_value"=w51, "magnets.elyse/magnets/Cor_V2/value"=w53) -> (w49:T5)
      n33 = local write "archive in"(w49) -> ()
    }
    frame #8 {
      n34 = Unbundle By Name(w60) -> ("31 ACH31 b66 Mes I correcte Dipôle 1 (H3)"=w59:dbl)
      n35 = Unbundle By Name(w58) -> ("04 OUT04 b17 Cmd Guidage H3"=w57:dbl)
      n36 = Bundle By Name(cluster=w56, "magnets.elyse/magnets/Cor_H3/set_value"=w57, "magnets.elyse/magnets/Cor_H3/value"=w59) -> (w55:T5)
      n37 = local write "archive in"(w55) -> ()
    }
    frame #9 {
      n38 = Unbundle By Name(w66) -> ("32 ACH32 b67 Mes I Guidage V3"=w65:dbl)
      n39 = Unbundle By Name(w64) -> ("05 OUT05 b21 Cmd Guidage V3"=w63:dbl)
      n40 = Bundle By Name(cluster=w62, "magnets.elyse/magnets/Cor_V3/set_value"=w63, "magnets.elyse/magnets/Cor_V3/value"=w65) -> (w61:T5)
      n41 = local write "archive in"(w61) -> ()
    }
    frame #10 {
      n42 = Unbundle By Name(w72) -> ("40 ACH40 b68 Mes I correcte Dipôle 21 (H4)"=w71:dbl)
      n43 = Unbundle By Name(w70) -> ("06 OUT06 b25 Cmd Guidage H4"=w69:dbl)
      n44 = Bundle By Name(cluster=w68, "magnets.elyse/magnets/Cor_H4/set_value"=w69, "magnets.elyse/magnets/Cor_H4/value"=w71) -> (w67:T5)
      n45 = local write "archive in"(w67) -> ()
    }
    frame #11 {
      n46 = Unbundle By Name(w78) -> ("33 ACH33 b69 Mes I Guidage V4"=w77:dbl)
      n47 = Unbundle By Name(w76) -> ("07 OUT07 b29 Cmd Guidage V4"=w75:dbl)
      n48 = Bundle By Name(cluster=w74, "magnets.elyse/magnets/Cor_V4/set_value"=w75, "magnets.elyse/magnets/Cor_V4/value"=w77) -> (w73:T5)
      n49 = local write "archive in"(w73) -> ()
    }
    frame #12 {
      n50 = Unbundle By Name(w84) -> ("34 ACH34 b71 Mes I Guidage V5"=w83:dbl)
      n51 = Unbundle By Name(w82) -> ("08 OUT08 b33 Réserve"=w81:dbl)
      n52 = Bundle By Name(cluster=w80, "magnets.elyse/magnets/Cor_H5/set_value"=w81, "magnets.elyse/magnets/Cor_H5/value"=w83) -> (w79:T5)
      n53 = local write "archive in"(w79) -> ()
    }
    frame #13 {
      n54 = Unbundle By Name(w87) -> ("34 ACH34 b71 Mes I Guidage V5"=w90:dbl)
      n55 = Unbundle By Name(w89) -> ("09 OUT09 b37 Cmd Guidage V5"=w88:dbl)
      n56 = Bundle By Name(cluster=w86, "magnets.elyse/magnets/Cor_V5/set_value"=w88, "magnets.elyse/magnets/Cor_V5/value"=w90) -> (w85:T5)
      n57 = local write "archive in"(w85) -> ()
    }
    frame #14 {
      n58 = Unbundle By Name(w93) -> ("00 OUT00 b01 Cmd I Triplet 1-1"=w94:dbl)
      n59 = Unbundle By Name(w96) -> ("16 ACH16 b51 Mes I Triplet 1-1"=w95:dbl)
      n60 = Bundle By Name(cluster=w92, "magnets.elyse/magnets/triplet1-1/set_value"=w94, "magnets.elyse/magnets/triplet1-1/value"=w95) -> (w91:T5)
      n61 = local write "archive in"(w91) -> ()
    }
    frame #15 {
      n62 = Unbundle By Name(w99) -> ("01 OUT01 b05 Cmd I Triplet 1-2"=w100:dbl)
      n63 = Unbundle By Name(w101) -> ("24 ACH24 b52 Mes I Triplet 1-2"=w102:dbl)
      n64 = Bundle By Name(cluster=w98, "magnets.elyse/magnets/triplet1-2/set_value"=w100, "magnets.elyse/magnets/triplet1-2/value"=w102) -> (w97:T5)
      n65 = local write "archive in"(w97) -> ()
    }
    frame #16 {
      n66 = Unbundle By Name(w107) -> ("03 OUT03 b13 Cmd I Triplet 2-1"=w106:dbl)
      n67 = Unbundle By Name(w108) -> ("25 ACH25 b54 Mes I Triplet 2-1"=w105:dbl)
      n68 = Bundle By Name(cluster=w104, "magnets.elyse/magnets/triplet2-1/set_value"=w106, "magnets.elyse/magnets/triplet2-1/value"=w105) -> (w103:T5)
      n69 = local write "archive in"(w103) -> ()
    }
    frame #17 {
      n70 = Unbundle By Name(w114) -> ("04 OUT04 b17 Cmd I Triplet 2-2"=w113:dbl)
      n71 = Unbundle By Name(w112) -> ("18 ACH18 b55 Mes I Triplet 2-2"=w111:dbl)
      n72 = Bundle By Name(cluster=w110, "magnets.elyse/magnets/triplet2-2/set_value"=w113, "magnets.elyse/magnets/triplet2-2/value"=w111) -> (w109:T5)
      n73 = local write "archive in"(w109) -> ()
    }
    frame #18 {
      n74 = Unbundle By Name(w120) -> ("19 ACH19 b57 Mes I Quadripôle 1"=w119:dbl)
      n75 = Unbundle By Name(w118) -> ("06 OUT06 b25 Cmd I Quad 1"=w117:dbl)
      n76 = Bundle By Name(cluster=w116, "magnets.elyse/magnets/qudrupole1/set_value"=w117, "magnets.elyse/magnets/qudrupole1/value"=w119) -> (w115:T5)
      n77 = local write "archive in"(w115) -> ()
    }
    frame #19 {
      n78 = Unbundle By Name(w126) -> ("27 ACH27 b58 Mes I Quadripôle 2"=w125:dbl)
      n79 = Unbundle By Name(w124) -> ("07 OUT07 b29 Cmd I Quad 2"=w123:dbl)
      n80 = Bundle By Name(cluster=w122, "magnets.elyse/magnets/qudrupole2/set_value"=w123, "magnets.elyse/magnets/qudrupole2/value"=w125) -> (w121:T5)
    }
  }
  "archive out" <- w1
